vi "Auton MaxTime.vi"(10 "MaxTime":dbl, 11 "Reset?":bool) -> (2 "Finished?":bool)   [LabVIEW 2016]
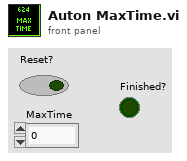
[diagram p1: front panel]
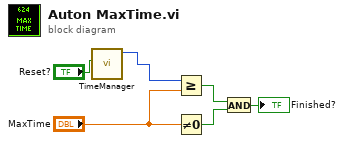
[diagram p0: block diagram]
diagram:
  n1 = call "TimeManager.vi"("Reset?"="Reset?") -> ("Time Since Reset"=w1:u32)  [unwired: 9 in, 1 out]
  n2 = Greater Or Equal?(x=w1, y="MaxTime") -> (x >= y?=w5:bool)
  n3 = Not Equal To 0?(x="MaxTime") -> (x != 0?=w4:bool)
  n4 = And(x=w5, y=w4) -> (x .and. y?=→"Finished?":bool)
